vi "Sine (Sub).vi"(4 "Sample":i32=10000, 5 "Time (s)":i32=10, 6 "Sine Frequency":dbl=200.0, 7 "File":path) -> (0 "Output Data":dbl[](array[numeric]), 1 "Waveform Graph":waveform(dbl)(graph))   [LabVIEW 2020]
uses:
  <vilib>/Analysis/NI_AALPro.lvlib
panel:
  out "Array Size":i32
  out "Data":dbl[](array[numeric])
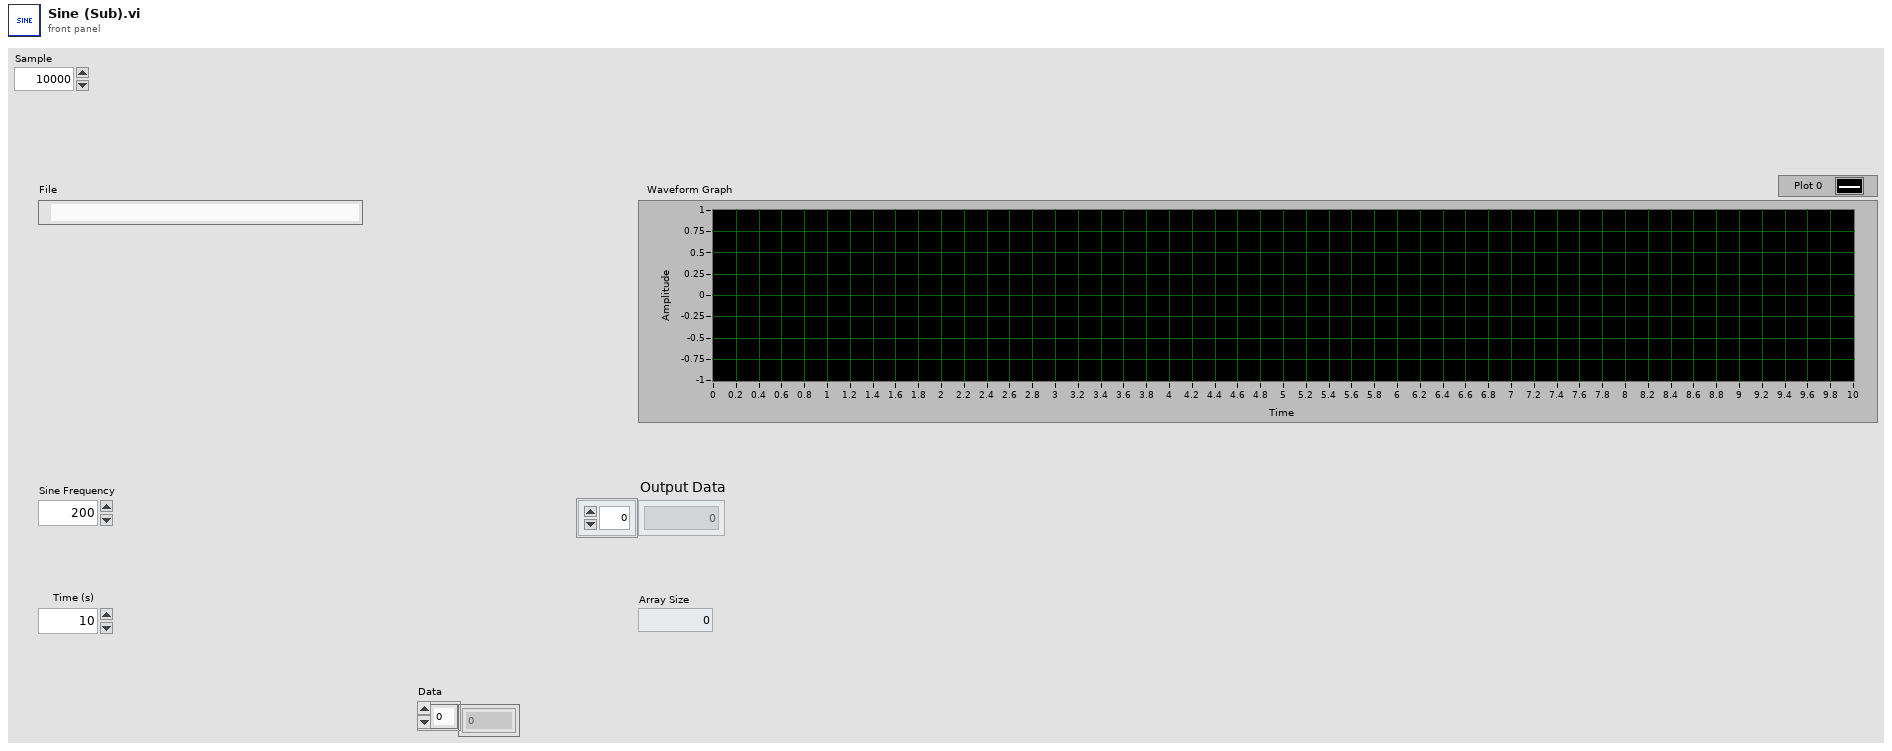
[diagram p1: front panel]
types:
  T1 = enum16{"sine", "cosine", "triangle", "square", "sawtooth", "increasing ramp", "decreasing ramp"}
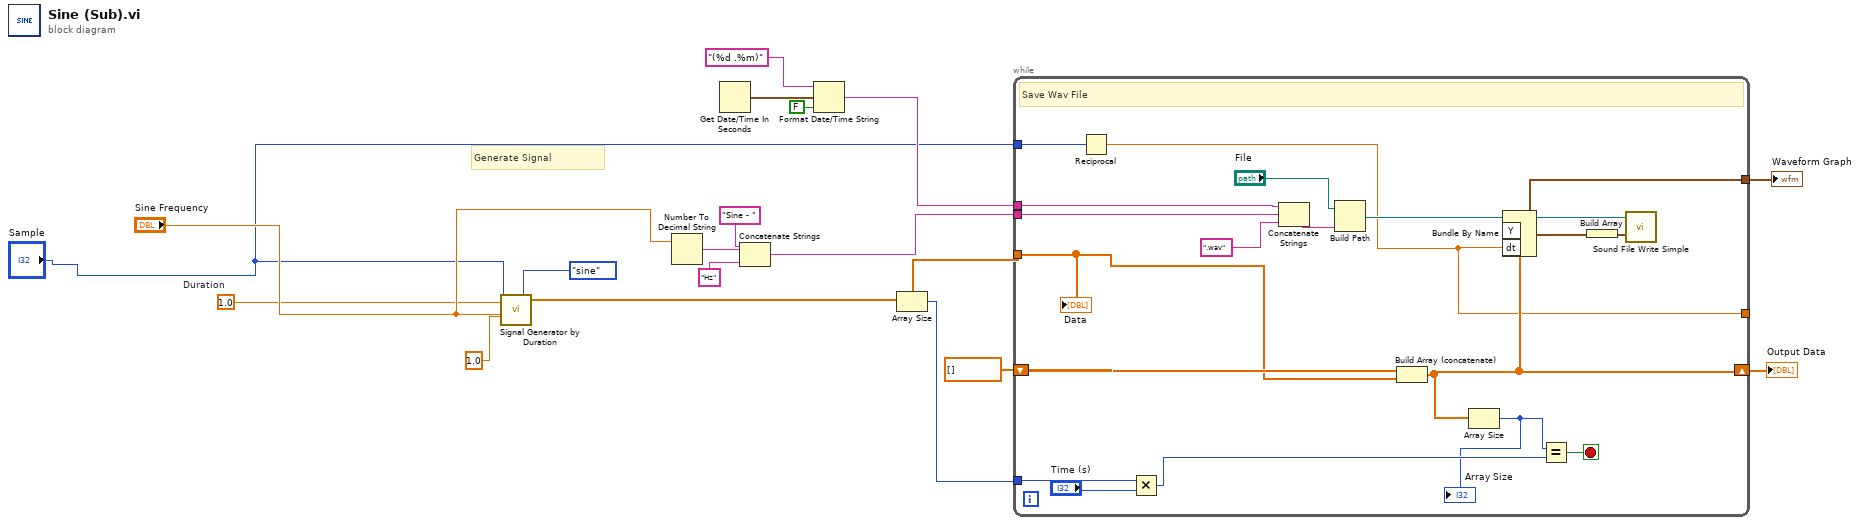
[diagram p0: block diagram]
diagram:
  w5 = 1.0  # Duration
  # "Generate Signal"
  n1 = call <vilib>:"Signal Generator by Duration.vi"("signal type"=T1."sine", "duration"=w5, "# of samples"="Sample", "frequency"="Sine Frequency", "amplitude"=1.0) -> ("signal"=w3:dbl[])  [unwired: 7 in, 3 out]
  n2 = Number To Decimal String(number="Sine Frequency") -> (decimal integer string=w18:string)  [unwired: 1 in]
  n3 = Get Date/Time In Seconds() -> (seconds since 1Jan1904=w10:timestamp)
  n4 = Concatenate Strings("Sine - ", w18, "Hz") -> (w9:string)
  n5 = Format Date/Time String(time format string (%c)="(%d .%m)", seconds (now)=w10, UTC format=FALSE) -> (date/time string=w13:string)
  n6 = Array Size(array=w3) -> (size(s)=w2:i32)
  n7 = while {
    tunnel: "Sample" -> [w36]
    tunnel: w3 -> [w33]
    shift-right: [w32] -> w8
    shift-left: dbl[] [] ("Array") -> [w34]
    tunnel: w2 -> [w28]
    tunnel: [w25] -> _
    tunnel: [w23] -> w7
    tunnel: w9 -> [w22]
    tunnel: w13 -> [w20]
    stop <- w31 stop-if-true
    # "Save Wav File"
    n8 = Reciprocal(x=w36) -> (1/x=w25:dbl)
    n9 = Multiply(x=w28, y="Time (s)") -> (x*y=w30:i32)
    n10 = Concatenate Strings(w20, w22, ".wav") -> (w24:string)
    n11 = Build Path(base path="File", name or relative path=w24) -> (appended path=w35:path)
    n12 = Build Array (concatenate)(w34, w33) -> (w32:dbl[])
    n13 = Array Size(array=w32) -> (size(s)=w29:i32)
    "Array Size" <- w29
    n14 = Bundle By Name("Y"=w32, "dt"=w25) -> (w23:waveform(dbl))  [unwired: 1 in]
    n15 = Equal?(x=w29, y=w30) -> (x = y?=w31:bool)
    n16 = Build Array(w23) -> (w26:waveform(dbl)[])
    n17 = call <vilib>:"Sound File Write Simple.vi"("data"=w26, "path"=w35) -> ()  [unwired: 8 in, 2 out]
    "Data" <- w33
  }
  "Output Data" <- w8
  "Waveform Graph" <- w7
